vi "Timer.vi"(8 "error constant":errorcluster, 10 "Reset":bool, 11 "Timing":u32) -> (0 "error constant 2":errorcluster, 1 "Time has Elapsed":bool, 3 "Numeric":dbl)   [LabVIEW 2016]
doc: "Return the elapsed time, and a boolean time elapsed when the sprinkle tine of the zone is reached."
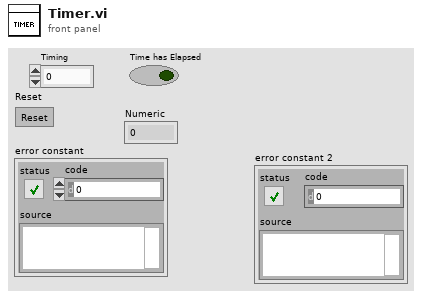
[diagram p1: front panel]
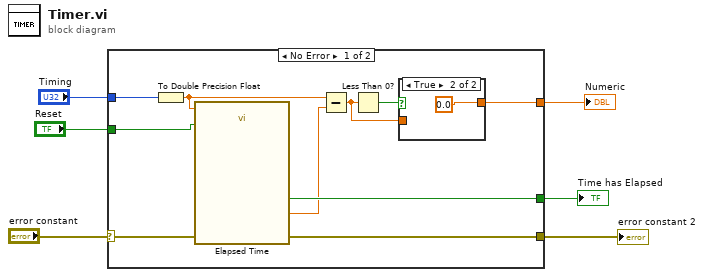
[diagram p0: block diagram]
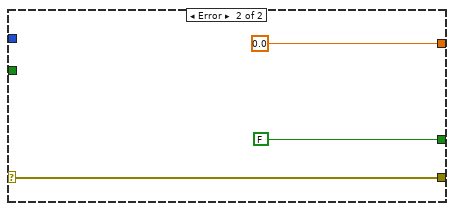
[diagram p3: hidden frame]
diagram:
  n1 = case shown="No Error" "error constant" {
    selector: "error constant" -> [w11 w20]
    tunnel: "Timing" -> [w15 _]
    tunnel: [w14 FALSE ("Time has Elapsed")] -> w5
    tunnel: [w9 0.0] -> w4
    tunnel: [w11 w20] -> w2
    tunnel: "Reset" -> [w7 _]
    frame No Error {
      n2 = To Double Precision Float(number=w15) -> (double precision float=w13:dbl)
      n3 = call "Elapsed Time"("Time Target (s)"=w13, "Reset"=w7) -> ("Elapsed Time (s)"=w12:dbl, "Time has Elapsed"=w14:bool)  [unwired: 10 in, 6 out]
      n4 = Subtract(x=w13, y=w12) -> (x-y=w8:dbl)
      n5 = Less Than 0?(x=w8) -> (x < 0?=w10:bool)
      n6 = case shown="True" w10 {
        tunnel: [w16 0.0] -> w9
        tunnel: w8 -> [w16 _]
        frame False {
        }
        frame True {
        }
      }
    }
    frame Error {
    }
  }
  "Time has Elapsed" <- w5
  "Numeric" <- w4
  "error constant 2" <- w2
